vi "speed average.vi"(0 "initialized array":dbl[][](array[numeric]), 5 "window size":i32, 7 "array speed in":dbl[](array[numeric])) -> (4 "1D array speed":dbl[](array[numeric]), 8 "2D average speed":dbl[][](array[numeric]))   [LabVIEW 2019]
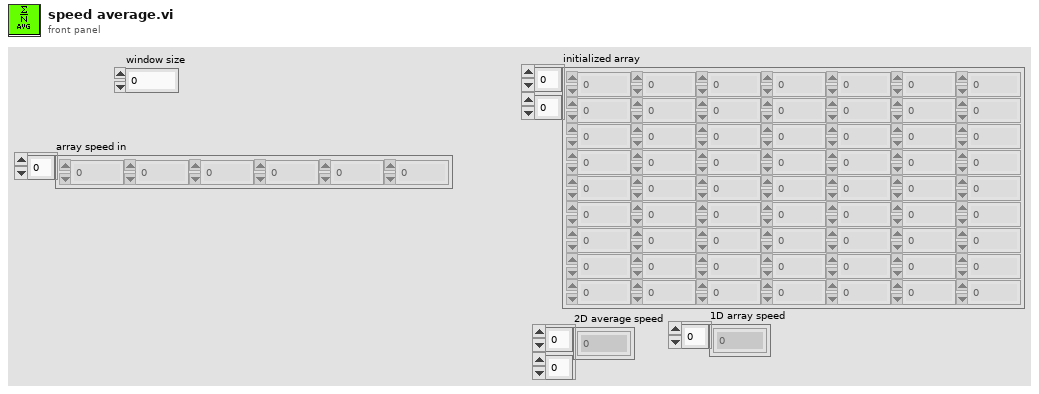
[diagram p1: front panel]
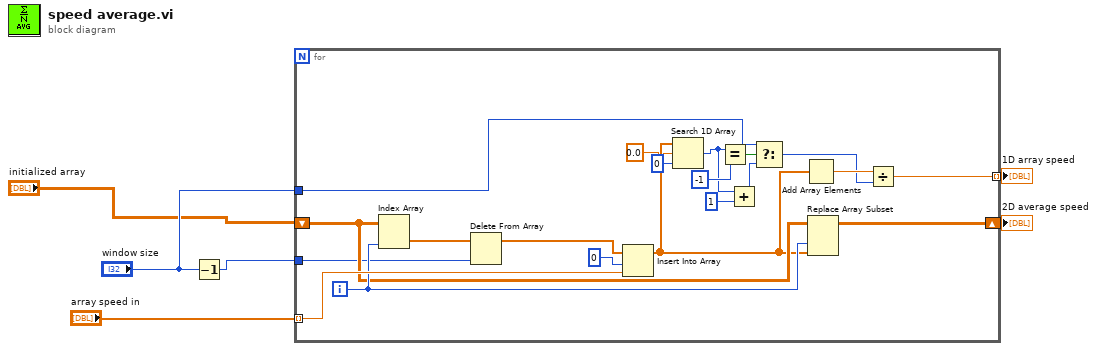
[diagram p0: block diagram]
diagram:
  n1 = Decrement(x="window size") -> (x-1=w6:i32)
  n2 = for {
    tunnel: "array speed in" -> [w22] mode=indexing
    tunnel: [w21] -> w1 mode=indexing
    shift-right: [w18] -> w2
    shift-left: "initialized array" -> [w19]
    tunnel: "window size" -> [w12]
    tunnel: w6 -> [w17]
    i -> [w20]
    n3 = Index Array "Index Array"(array=w19, index (col)=w20) -> (element=w25:dbl[])  [unwired: 1 in]
    n4 = Delete From Array "Delete From Array"(array=w25, index=w17) -> (array with subset deleted=w24:dbl[])  [unwired: 1 in, 1 out]
    n5 = Insert Into Array "Insert Into Array"(array=w24, index=0, new element=w22) -> (w16:dbl[])
    n6 = Search 1D Array(1D array=w16, element=0.0, start index (0)=0) -> (index of element=w9:i32)
    n7 = Equal?(x=w9, y=-1) -> (x = y?=w14:bool)
    n8 = Add(x=w9, y=1) -> (x+y=w7:i32)
    n9 = Select(t=w12, s=w14, f=w7) -> (s? t:f=w11:i32)
    n10 = Add Array Elements(numeric array=w16) -> (sum=w23:dbl)
    n11 = Replace Array Subset "Replace Array Subset"(array=w19, new element=w16, index (col)=w20) -> (w18:dbl[][])  [unwired: 1 in]
    n12 = Divide(x=w23, y=w11) -> (x/y=w21:dbl)
  }
  "2D average speed" <- w2
  "1D array speed" <- w1
